vi "光标.vi"(8 "错误输入":errorcluster caption="错误输入（无错误）", 11 "引用":refnum<k24>) -> (0 "错误输出":errorcluster, 3 "引用输出":refnum<k24>)   [LabVIEW 2018]
uses:
  ScintillaNET.dll
  System.Drawing
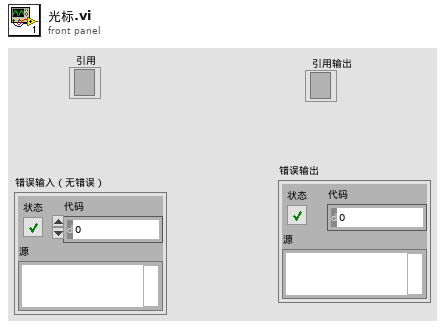
[diagram p1: front panel]
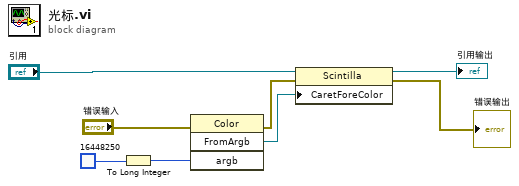
[diagram p0: block diagram]
diagram:
  n1 = To Long Integer(number=u32 16448250 ("前景色")) -> (32bit integer=w8:i32)
  n2 = invoke class="Color" method="FromArgb"(error in="错误输入", "argb"=w8) -> (error out=w2:errorcluster, "FromArgb"=w6:refnum<k24>)  [unwired: 2 in, 2 out]
  n3 = property class="Scintilla"(reference="引用", error in=w2, "CaretForeColor"=w6) -> (reference out=→"引用输出":refnum<k24>, error out=→"错误输出":errorcluster)
